vi "LPS22HH.vi"() -> ()   [LabVIEW 2020, in "LPS22Demo.lvlib"]
uses:
  <instrlib>/niDigital/niDigital.llb/niDigital Data Mapping.ctl
  <instrlib>/niDigital/niDigital.llb/niDigital Bit Order.ctl
  <instrlib>/niDigital/niDigital.llb/niDigital Create Source Waveform (Serial).vi
  <instrlib>/niDigital/niDigital.llb/niDigital Create Capture Waveform (Parallel).vi
  <instrlib>/niDigital/niDigital.llb/niDigital Write Source Waveform (Broadcast U32).vi
  <instrlib>/niDigital/niDigital.llb/niDigital Burst Pattern (Burst Only).vi
  LPS22Demo.lvlib
panel:
  out "Thermometer":dbl(slide) scale=0.0..40.0
  out "Data":bool[](array[boolean])
  out "R/W":bool
  out "Address":bool[](array[boolean])
  out "RX data":u32[](array[numeric])
  in  "stop":bool
  in  "Burst":bool
  in  "DUT power up/down":bool=TRUE
  in  "Write Data":i8 format="%.0b"
  in  "Register":u16(ring)=15 items=["INTERRUPT_CFG"=11, "THS_P_L"=12, "THS_P_H"=13, "IF_CTRL"=14, "WHO_AM_I"=15, "CTRL_REG1"=16, "CTRL_REG2"=17, "CTRL_REG3"=18, "FIFO_CTRL"=19, "FIFO_WTM"=20, "RPDS_L"=24, "RPDS_H"=25, "INT_SOURCE"=36, "FIFO_STATUS1"=37, "FIFO_STATUS2"=38, "STATUS"=39, "PRESSURE_OUT_XL"=40, "PRESSURE_OUT_L"=41, "PRESSURE_OUT_H"=42, "TEMP_OUT_L"=43, "TEMP_OUT_H"=44, "FIFO_DATA_OUT_PRESS_XL"=120, "FIFO_DATA_OUT_PRESS_L"=121, "FIFO_DATA_OUT_PRESS_H"=122, "FIFO_DATA_OUT_TEMP_L"=123, "FIFO_DATA_OUT_TEMP_H"=124]
  in  "Read/Write":i16(ring)=1 items=["Write", "Read"]
  in  "resource name":refnum<k15>="S5_6570"
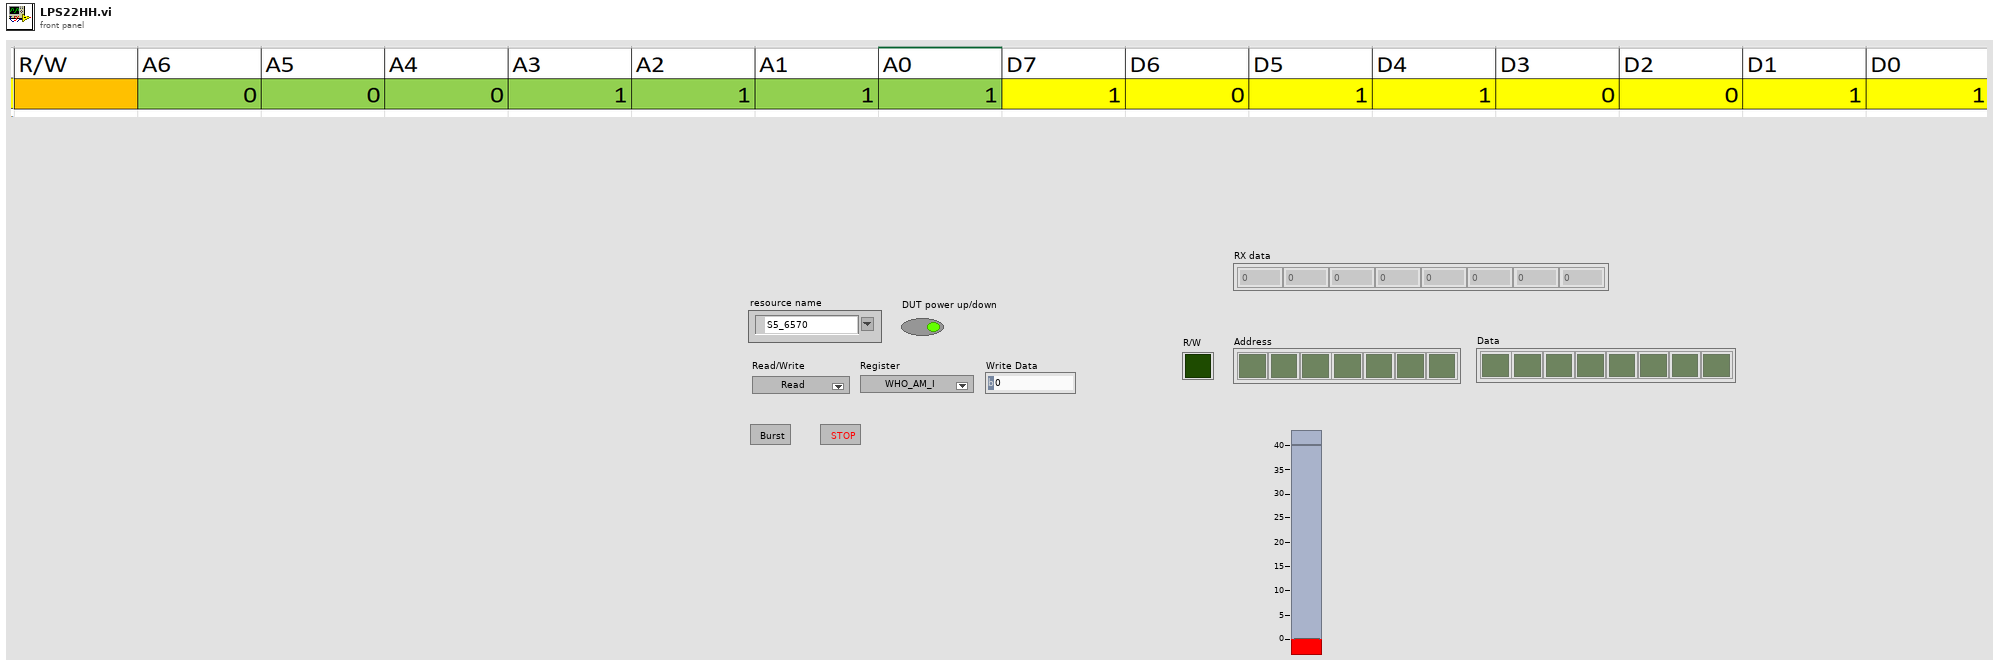
[diagram p1: front panel]
types:
  T1 = typedef "niDigital Bit Order.ctl" = i32
  T2 = typedef "niDigital Data Mapping.ctl" = i32
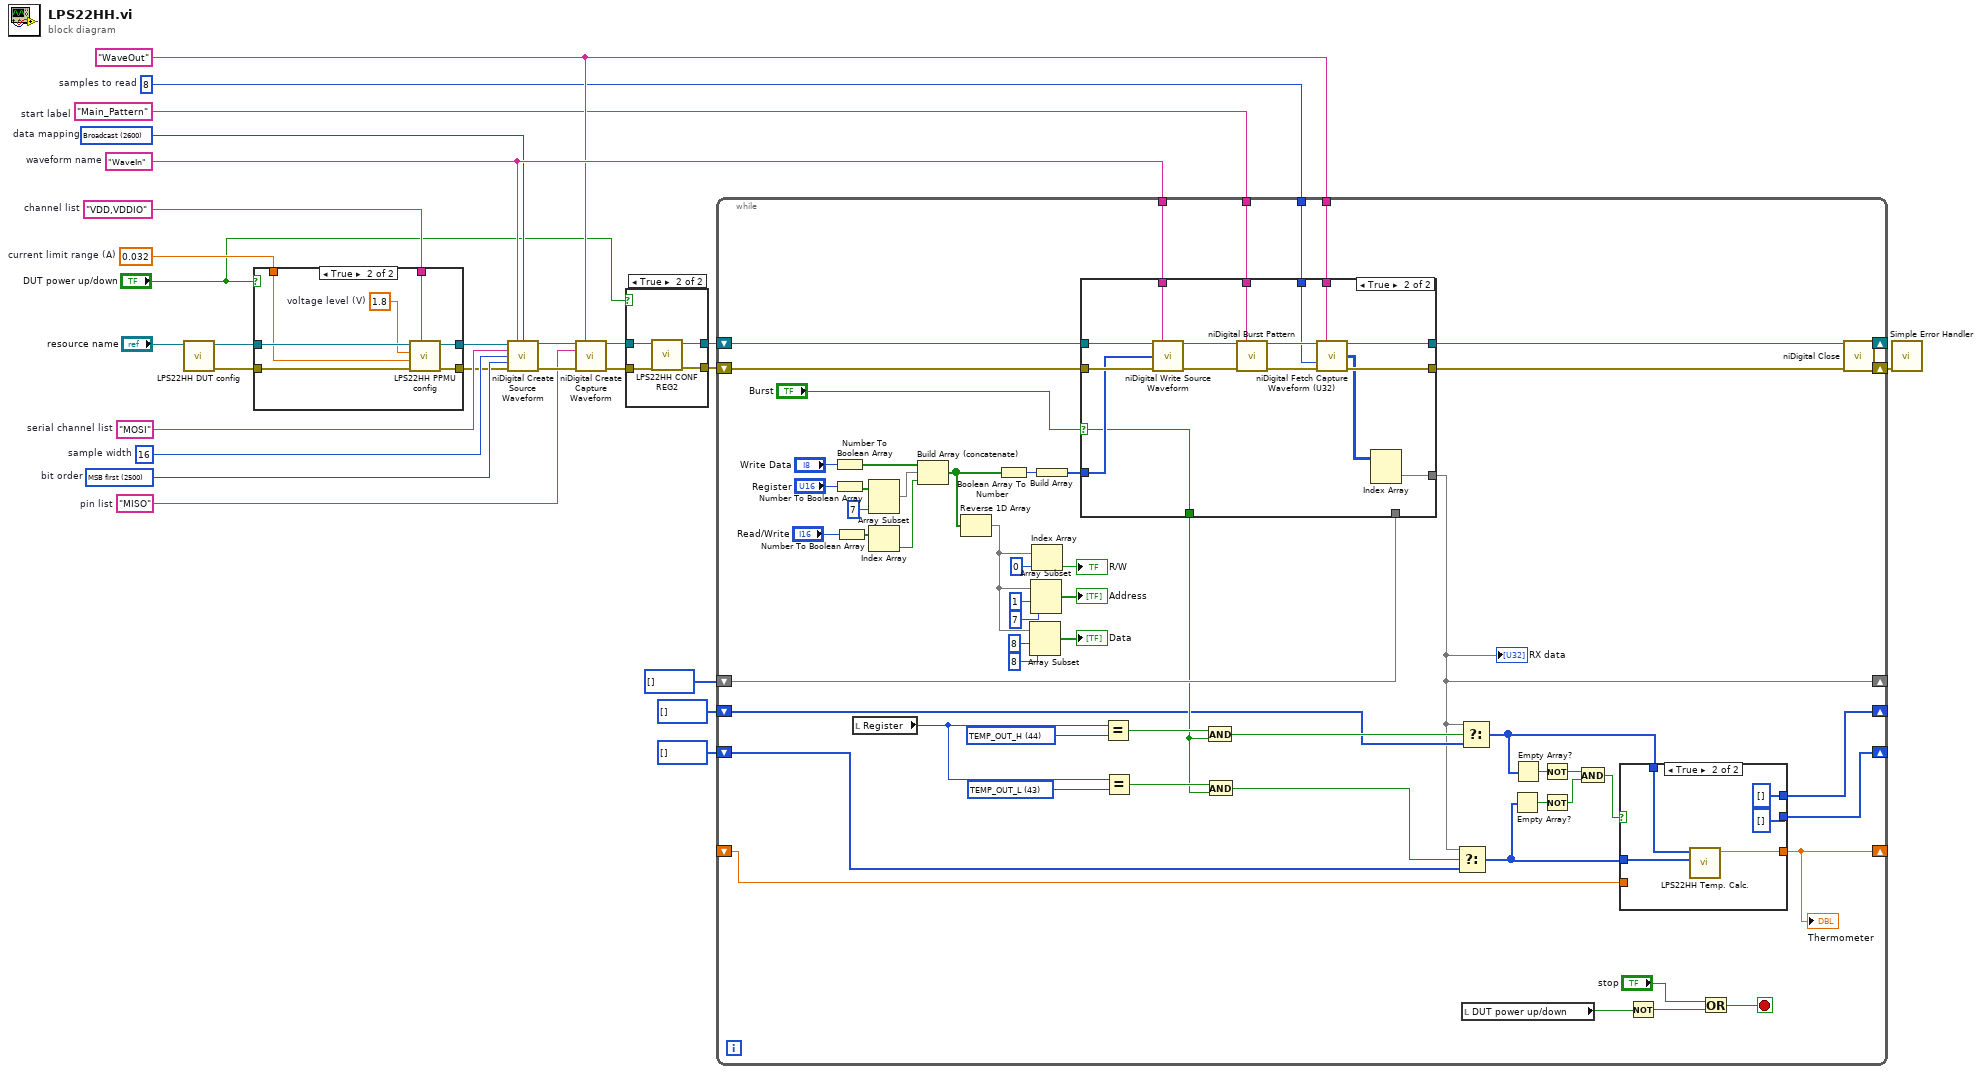
[diagram p0: block diagram]
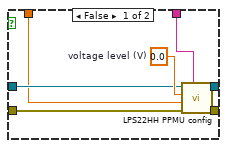
[diagram p5: hidden frame]
diagram:
  w9 = 8  # samples to read
  w10 = "Main_Pattern"  # start label
  w13 = 0.032  # current limit range (A)
  w14 = "VDD,VDDIO"  # channel list
  w19 = "MISO"  # pin list
  w18 = "WaveOut" ("waveform name")
  w27 = "MOSI"  # serial channel list
  w26 = u32 16  # sample width
  w24 = T1 2500 items=["MSB first"=2500, "LSB first"=2501]  # bit order
  w25 = T2 2600 items=["Broadcast"=2600, "Site Unique"=2601]  # data mapping
  w28 = "WaveIn"  # waveform name
  n1 = call "LPS22HH DUT config.vi"("resource name"="resource name") -> ("error out"=w15:errorcluster, "instrument handle out"=w16:refnum<k15>)  [unwired: 7 in]
  n2 = case shown="True" "DUT power up/down" {
    tunnel: w16 -> [w33 w43]
    tunnel: w15 -> [w35 w42]
    tunnel: w14 -> [w31 w41]
    tunnel: w13 -> [w30 w40]
    tunnel: [w32 w38] -> w12
    tunnel: [w34 w37] -> w11
    frame False {
      w36 = 0.0  # voltage level (V)
      n3 = call "LPS22HH PPMU config.vi"("channel list"=w31, "error in"=w35, "current limit range (A)"=w30, "voltage level (V)"=w36, "instrument handle"=w33) -> ("error out"=w34:errorcluster, "instrument handle out"=w32:refnum<k15>)  [unwired: 5 in]
    }
    frame True {
      w39 = 1.8  # voltage level (V)
      n4 = call "LPS22HH PPMU config.vi"("channel list"=w41, "error in"=w42, "current limit range (A)"=w40, "voltage level (V)"=w39, "instrument handle"=w43) -> ("error out"=w37:errorcluster, "instrument handle out"=w38:refnum<k15>)  [unwired: 5 in]
    }
  }
  n5 = call-poly <instrlib>:"niDigital Create Source Waveform.vi"("instrument handle"=w12, "waveform name"=w28, "data mapping"=w25, "pin list"=w27, "sample width"=w26, "bit order"=w24, "error in"=w11) -> ("instrument handle out"=w22:refnum<k15>, "error out"=w23:errorcluster)  [unwired: 7 in]
  n6 = call-poly <instrlib>:"niDigital Create Capture Waveform.vi"("instrument handle"=w22, "waveform name"=w18, "pin list"=w19, "error in"=w23) -> ("instrument handle out"=w4:refnum<k15>, "error out"=w7:errorcluster)  [unwired: 10 in]
  n7 = case shown="True" "DUT power up/down" {
    tunnel: w7 -> [w44 w49]
    tunnel: [w44 w48] -> w6
    tunnel: [w45 w47] -> w5
    tunnel: w4 -> [w45 w46]
    frame False {
    }
    frame True {
      n8 = call "LPS22HH CONF REG2.vi"("error in"=w49, "instrument handle"=w46) -> ("error out"=w48:errorcluster, "instrument handle out"=w47:refnum<k15>)  [unwired: 8 in]
    }
  }
  n9 = while {
    tunnel: w28 -> [w106]
    tunnel: w18 -> [w101]
    tunnel: w10 -> [w100]
    tunnel: w9 -> [w99]
    shift-right: [w102] -> w20
    shift-left: w6 -> [w105]
    shift-right: [w103] -> w21
    shift-left: w5 -> [w104]
    shift-right: [w62] -> _
    shift-left: u32[] [] ("data") -> [w87]
    shift-right: [w50] -> _
    shift-left: u32[] [] ("data") -> [w64]
    shift-right: [w51] -> _
    shift-left: u32[] [] ("data") -> [w61]
    shift-right: [w52] -> _
    shift-left: _ -> [w53]
    stop <- w85 stop-if-true
    w71 = u16 43 items=["INTERRUPT_CFG"=11, "THS_P_L"=12, "THS_P_H"=13, "IF_CTRL"=14, "WHO_AM_I"=15, "CTRL_REG1"=16, "CTRL_REG2"=17, "CTRL_REG3"=18, "FIFO_CTRL"=19, "FIFO_WTM"=20, "RPDS_L"=24, "RPDS_H"=25, "INT_SOURCE"=36, "FIFO_STATUS1"=37, "FIFO_STATUS2"=38, "STATUS"=39, "PRESSURE_OUT_XL"=40, "PRESSURE_OUT_L"=41, "PRESSURE_OUT_H"=42, "TEMP_OUT_L"=43, "TEMP_OUT_H"=44, "FIFO_DATA_OUT_PRESS_XL"=120, "FIFO_DATA_OUT_PRESS_L"=121, "FIFO_DATA_OUT_PRESS_H"=122, "FIFO_DATA_OUT_TEMP_L"=123, "FIFO_DATA_OUT_TEMP_H"=124] ("Register 2")
    w72 = u16 44 items=["INTERRUPT_CFG"=11, "THS_P_L"=12, "THS_P_H"=13, "IF_CTRL"=14, "WHO_AM_I"=15, "CTRL_REG1"=16, "CTRL_REG2"=17, "CTRL_REG3"=18, "FIFO_CTRL"=19, "FIFO_WTM"=20, "RPDS_L"=24, "RPDS_H"=25, "INT_SOURCE"=36, "FIFO_STATUS1"=37, "FIFO_STATUS2"=38, "STATUS"=39, "PRESSURE_OUT_XL"=40, "PRESSURE_OUT_L"=41, "PRESSURE_OUT_H"=42, "TEMP_OUT_L"=43, "TEMP_OUT_H"=44, "FIFO_DATA_OUT_PRESS_XL"=120, "FIFO_DATA_OUT_PRESS_L"=121, "FIFO_DATA_OUT_PRESS_H"=122, "FIFO_DATA_OUT_TEMP_L"=123, "FIFO_DATA_OUT_TEMP_H"=124] ("Register 2")
    n10 = Number To Boolean Array(number="Write Data") -> (Boolean array=w97:bool[])
    n11 = Number To Boolean Array(number="Register") -> (Boolean array=w93:bool[])
    n12 = Number To Boolean Array(number="Read/Write") -> (Boolean array=w92:bool[])
    n13 = local read "Register"() -> (w69:u16)
    n14 = Array Subset(array=w93, length=7) -> (w94:bool[])  [unwired: 1 in]
    n15 = Index Array(array=w92) -> (element=w95:bool)  [unwired: 1 in]
    n16 = Build Array (concatenate)(w97, w94, w95) -> (w74:bool[])
    n17 = Reverse 1D Array(array=w74) -> (reversed array=w73:bool[])
    n18 = Boolean Array To Number(Boolean array=w74) -> (number=w98:u32)
    n19 = Array Subset(array=w73, index=8, length=8) -> (→"Data":bool[])
    n20 = Array Subset(array=w73, index=1, length=7) -> (→"Address":bool[])
    n21 = Index Array(array=w73, index=0) -> (element=→"R/W":bool)
    n22 = Build Array(w98) -> (w89:u32[])
    n23 = case shown="True" "Burst" {
      selector: "Burst" -> [w115 w119]
      tunnel: w106 -> [_ w134]
      tunnel: w105 -> [w118 w133]
      tunnel: w104 -> [w117 w132]
      tunnel: [w117 w131] -> w103
      tunnel: [w118 w130] -> w102
      tunnel: w101 -> [_ w129]
      tunnel: w100 -> [_ w128]
      tunnel: w99 -> [_ w123]
      tunnel: w89 -> [_ w121]
      tunnel: [w116 w120] -> w62
      tunnel: w87 -> [w116 _]
      tunnel: [w115 w119] -> w66
      frame False {
      }
      frame True {
        n24 = call-poly <instrlib>:"niDigital Write Source Waveform.vi"("instrument handle"=w132, "waveform name"=w134, "waveform data"=w121, "error in"=w133) -> ("instrument handle out"=w126:refnum<k15>, "error out"=w127:errorcluster)  [unwired: 10 in]
        n25 = call-poly <instrlib>:"niDigital Burst Pattern.vi"("instrument handle"=w126, "start label"=w128, "error in"=w127) -> ("instrument handle out"=w125:refnum<k15>, "error out"=w124:errorcluster)  [unwired: 11 in]
        n26 = call <instrlib>:"niDigital Fetch Capture Waveform (U32).vi"("instrument handle"=w125, "waveform name"=w129, "samples to read"=w123, "error in"=w124) -> ("instrument handle out"=w131:refnum<k15>, "data"=w122:u32[][], "error out"=w130:errorcluster)  [unwired: 9 in]
        n27 = Index Array(array=w122) -> (element=w120:u32[])  [unwired: 2 in]
      }
    }
    "RX data" <- w62
    n28 = Equal?(x=w69, y=w72) -> (x = y?=w67:bool)
    n29 = Equal?(x=w69, y=w71) -> (x = y?=w68:bool)
    n30 = And(x=w67, y=w66) -> (x .and. y?=w65:bool)
    n31 = And(x=w68, y=w66) -> (x .and. y?=w63:bool)
    n32 = Select(t=w62, s=w63, f=w61) -> (s? t:f=w54:u32[])
    n33 = Select(t=w62, s=w65, f=w64) -> (s? t:f=w55:u32[])
    n34 = local read "DUT power up/down"() -> (w84:bool)
    n35 = Empty Array?(array=w54) -> (empty?=w59:bool)
    n36 = Empty Array?(array=w55) -> (empty?=w60:bool)
    n37 = Not(x=w60) -> (.not. x?=w58:bool)
    n38 = Not(x=w59) -> (.not. x?=w57:bool)
    n39 = And(x=w58, y=w57) -> (x .and. y?=w56:bool)
    n40 = case shown="True" w56 {
      tunnel: w55 -> [w107 w114]
      tunnel: w54 -> [w108 w113]
      tunnel: [w109 w112] -> w52
      tunnel: w53 -> [w109 _]
      tunnel: [w108 u32[] [] ("data")] -> w51
      tunnel: [w107 u32[] [] ("data")] -> w50
      frame False {
      }
      frame True {
        n41 = call "LPS22HH Temp. Calc..vi"("TEMP_OUT_L"=w113, "TEMP_OUT_H"=w114) -> ("Thermometer"=w112:dbl)  [unwired: 9 in]
      }
    }
    "Thermometer" <- w52
    n42 = Not(x=w84) -> (.not. x?=w83:bool)
    n43 = Or(x="stop", y=w83) -> (x .or. y?=w85:bool)
  }
  n44 = call <instrlib>:"niDigital Close.vi"("instrument handle"=w21, "error in"=w20) -> ("error out"=w29:errorcluster)  [unwired: 13 in]
  n45 = call <vilib>:"Simple Error Handler.vi"("error in (no error)"=w29) -> ()  [unwired: 4 in, 5 out]
